vi "View Next Tab.vi"(7 "QRD":T1, 8 "error in":errorcluster) -> (0 "error out":errorcluster, 5 "QRD Out":T1)   [LabVIEW 2025]
uses:
  Controls/Queues-Refs-Data.ctl
  Builds/Queue Wrappers.lvlibp/Q Packet.ctl
  Builds/Queue Wrappers.lvlibp
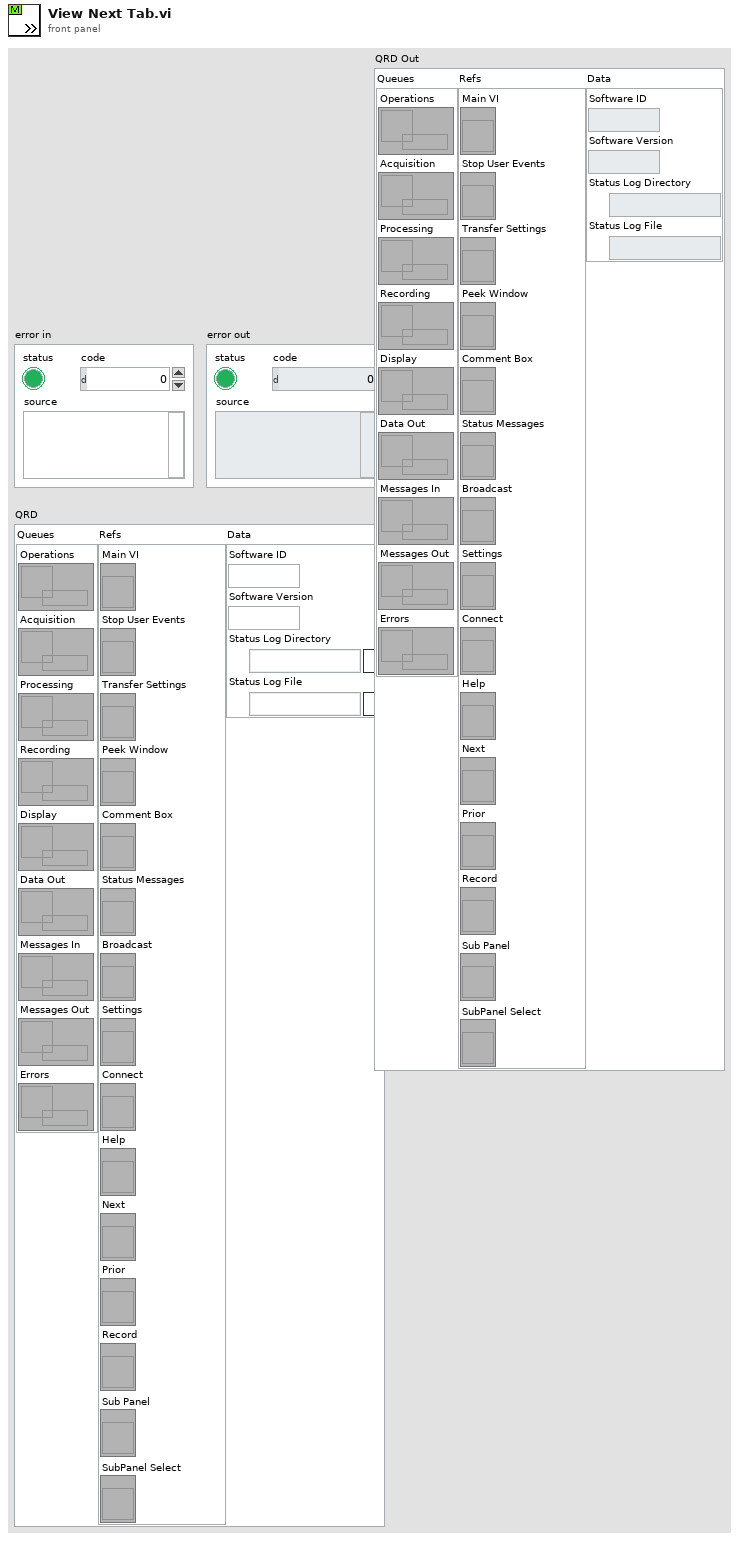
[diagram p1: front panel]
types:
  T1 = typedef "Queues-Refs-Data.ctl" = cluster{"Queues":cluster{"Operations":refnum<queue>, "Acquisition":refnum<queue>, "Processing":refnum<queue>, "Recording":refnum<queue>, "Display":refnum<queue>, "Data Out":refnum<queue>, "Messages In":refnum<queue>, "Messages Out":refnum<queue>, "Errors":refnum<queue>}, "Refs":cluster{"Main VI":refnum<vi>, "Stop User Events":refnum<vi>, "Transfer Settings":refnum<vi>, "Peek Window":refnum<vi>, "Comment Box":refnum<vi>, "Status Messages":refnum<vi>, "Broadcast":refnum<vi>, "Settings":refnum<vi>, "Connect":refnum<vi>, "Help":refnum<vi>, "Next":refnum<vi>, "Prior":refnum<vi>, "Record":refnum<vi>, "Sub Panel":refnum<vi>, "SubPanel Select":refnum<vi>}, "Data":cluster{"Software ID":string, "Software Version":string, "Status Log Directory":path, "Status Log File":path}}
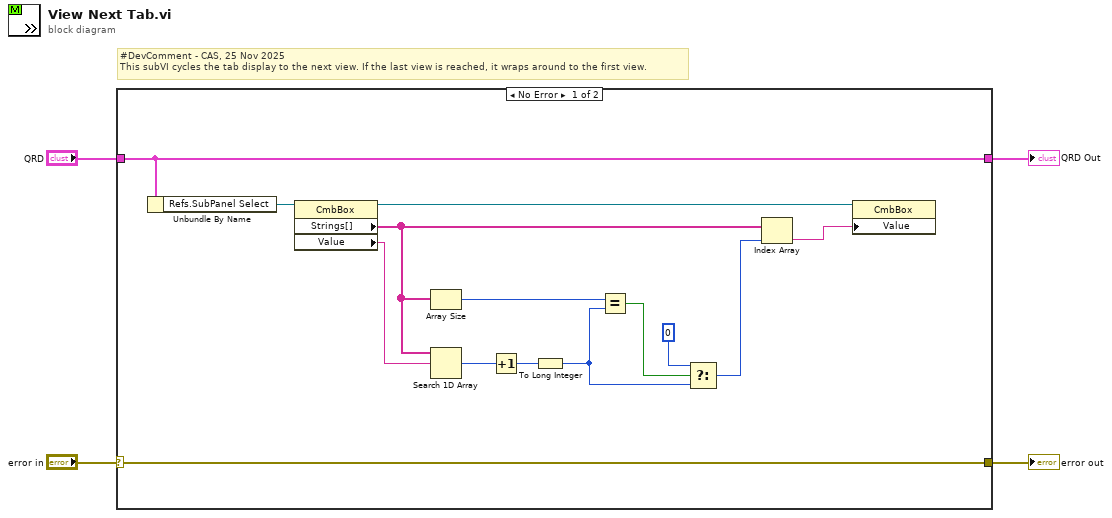
[diagram p0: block diagram]
diagram:
  # "#DevComment - CAS, 25 Nov 2025\nThis subVI cycles the tab display to the next view. If the last view is reached, it wraps around to the first view."
  n1 = case shown="No Error" "error in" {
    selector: "error in" -> [w5 w19]
    tunnel: [w5 w19] -> w3
    tunnel: "QRD" -> [w11 w20]
    tunnel: [w11 w20] -> w1
    frame No Error {
      n2 = Unbundle By Name(w11) -> ("Refs.SubPanel Select"=w18:refnum<vi>)
      n3 = property class="CmbBox"(reference=w18) -> (reference out=w17:refnum<vi>, "Strings[]"=w8:string[], "Value"=w7:string)  [unwired: 1 in, 1 out]
      n4 = Array Size(array=w8) -> (size(s)=w16:i32)
      n5 = Search 1D Array(1D array=w8, element=w7) -> (index of element=w6:i32)  [unwired: 1 in]
      n6 = Increment(x=w6) -> (x+1=w15:i32)
      n7 = To Long Integer(number=w15) -> (32bit integer=w13:i32)
      n8 = Equal?(x=w16, y=w13) -> (x = y?=w14:bool)
      n9 = Select(t=0, s=w14, f=w13) -> (s? t:f=w9:i32)
      n10 = Index Array(array=w8, index=w9) -> (element=w10:string)
      n11 = property class="CmbBox"(reference=w17, "Value"=w10) -> ()  [unwired: 1 in, 2 out]
    }
    frame Error {
    }
  }
  "error out" <- w3
  "QRD Out" <- w1
